vi "Cleanup GObject DB.vi"(8 "error in (no error)":errorcluster, 11 "Project Data in":refnum<class "Project Data.lvclass">) -> (0 "error out":errorcluster, 3 "Project Data out":refnum<class "Project Data.lvclass">)   [LabVIEW 2013, in "SET Project Data.lvlib" / "Project Data.lvclass"]
uses:
  Project Data.lvclass
  Project Data.lvclass/Project Data.ctl
  VI Class/VI Data.lvclass
  Menu Class/Menu Data.lvclass/Menu Data.ctl
  Menu Class/Read Menu Path (Relative).vi
  Menu Class/Menu Data.lvclass
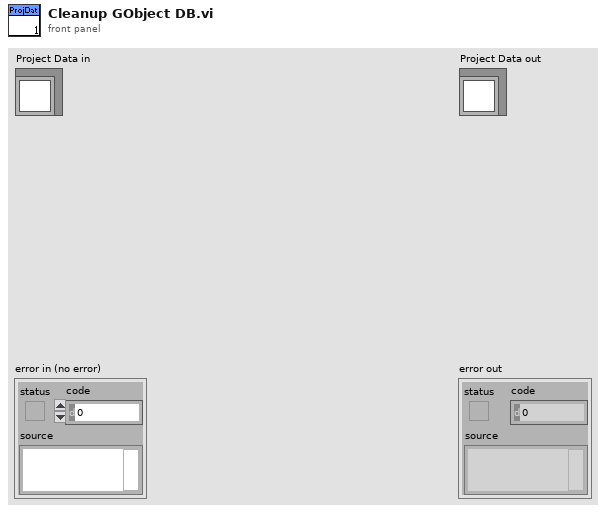
[diagram p1: front panel]
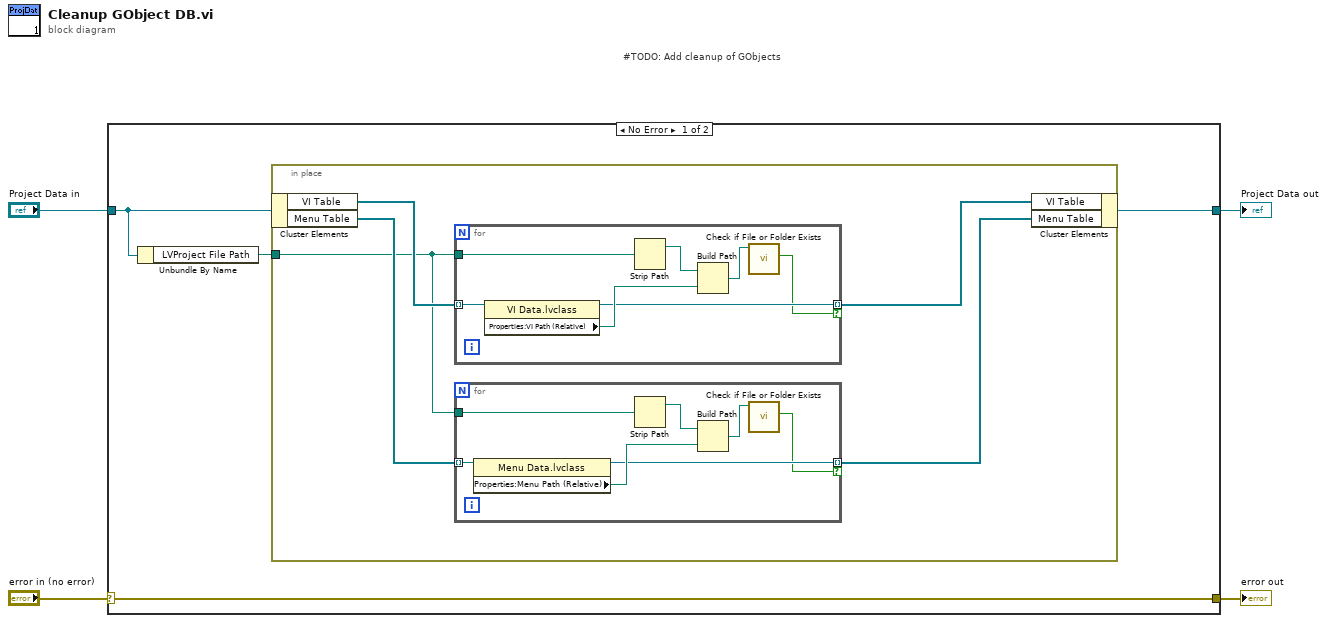
[diagram p0: block diagram]
diagram:
  # "#TODO: Add cleanup of GObjects"
  n1 = case shown="No Error" "error in (no error)" {
    selector: "error in (no error)" -> [w5 w29]
    tunnel: [w5 w29] -> w3
    tunnel: [w6 w28] -> w1
    tunnel: "Project Data in" -> [w8 w28]
    frame No Error {
      n2 = Unbundle By Name(w8) -> ("LVProject File Path"=w7:path)
      n3 = in-place {
        in-place-border: w7 -> [w9]
        n4 = in-place-cluster #1(w8) -> ("VI Table"=w13:refnum<class "VI Data.lvclass">[], "Menu Table"=w12:refnum<class "Menu Data.lvclass">[])
        n5 = for {
          tunnel: w13 -> [w27] mode=indexing
          tunnel: w9 -> [w25]
          tunnel: [w22] -> w11 mode=indexing if=w21
          n6 = property class="VI Data.lvclass"(reference=w27) -> (reference out=w22:refnum<class "VI Data.lvclass">, "Properties:VI Path (Relative)"=w24:path)  [unwired: 1 in, 1 out]
          n7 = Strip Path(path=w25) -> (stripped path=w26:path)  [unwired: 1 out]
          n8 = Build Path(base path=w26, name or relative path=w24) -> (appended path=w23:path)
          n9 = call <vilib>:"Check if File or Folder Exists.vi"("path"=w23) -> ("file or folder exists?"=w21:bool)  [unwired: 8 in, 2 out]
        }
        n10 = for {
          tunnel: w12 -> [w20] mode=indexing
          tunnel: w9 -> [w18]
          tunnel: [w15] -> w10 mode=indexing if=w14
          n11 = property class="Menu Data.lvclass"(reference=w20) -> (reference out=w15:refnum<class "Menu Data.lvclass">, "Properties:Menu Path (Relative)"=w17:path)  [unwired: 1 in, 1 out]
          n12 = Strip Path(path=w18) -> (stripped path=w19:path)  [unwired: 1 out]
          n13 = Build Path(base path=w19, name or relative path=w17) -> (appended path=w16:path)
          n14 = call <vilib>:"Check if File or Folder Exists.vi"("path"=w16) -> ("file or folder exists?"=w14:bool)  [unwired: 8 in, 2 out]
        }
        n15 = in-place-cluster #1("VI Table"=w11, "Menu Table"=w10) -> (w6:refnum<class "Project Data.lvclass">)
      }
    }
    frame Error {
    }
  }
  "error out" <- w3
  "Project Data out" <- w1
